vi "DAQmx_Pulse_TrainSlow.vi"(0 "Counter(s)":tag="PXI1Slot3/ctr1", 1 "Start?":bool=TRUE, 3 "FillTime":dbl=20.0 format="%0.2f", 5 "DrainTime":dbl=1.0 min=0.0 format="%0.2f") -> ()   [LabVIEW 2011]
doc: "This VI is set to drive a \"puffer\" valve for pulsed gas releases. It is configured for the stack to be connected to the Normally Open valve port (oddly!)- this is because that port was found to permit higher flow rates. The default logic level has been adjusted accordingly."
uses:
  <vilib>/DAQmx/create/channels.llb/DAQmx Create Channel (CO-Pulse Generation-Time).vi
  <vilib>/DAQmx/configure/timing.llb/DAQmx Timing (Implicit).vi
panel:
  out "error out":errorcluster
  # "For instructions, select Help>>Show Context Help"
  # "Channel Parameters"
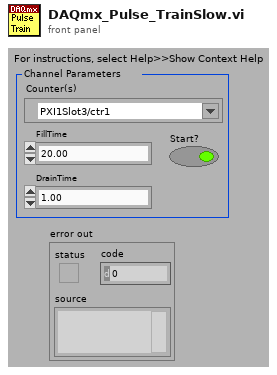
[diagram p1: front panel]
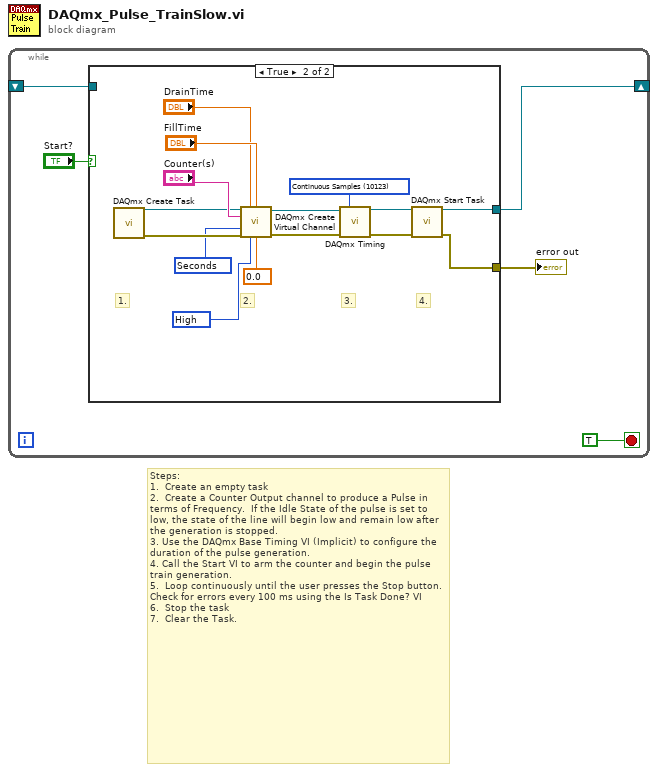
[diagram p0: block diagram]
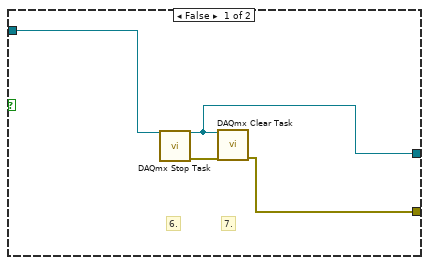
[diagram p2: hidden frame]
diagram:
  # "Steps: \n1.  Create an empty task\n2.  Create a Counter Output channel to produce a Pulse in terms of Frequency.  If the Idle State of the pulse is set to low, the state of the line will begin low and remain low after the generation is stopped.\n3. Use the DAQmx Base Timing VI (Implicit) to configure the duration of the pulse generation.\n4. Call the Start VI to arm the counter and begin the pulse train generation.\n5.  Loop continuously until the user presses the Stop button. Check for errors every 100 ms using the Is Task Done? VI\n6.  Stop the task\n7.  Clear the Task."
  n1 = while {
    shift-right: [w5] -> _
    shift-left: _ -> [w3]
    stop <- TRUE stop-if-true
    n2 = case shown="True" "Start?" {
      tunnel: [w7 w15] -> w5
      tunnel: w3 -> [w8 _]
      tunnel: [w6 w12] -> w1
      frame False {
        # "7."
        # "6."
        n3 = call <vilib>:"DAQmx Stop Task.vi"("task/channels in"=w8) -> ("task out"=w7:refnum<k21>, "error out"=w9:errorcluster)  [unwired: 1 in, 12 out]
        n4 = call <vilib>:"DAQmx Clear Task.vi"("task in"=w7, "error in"=w9) -> ("error out"=w6:errorcluster)  [unwired: 13 out]
      }
      frame True {
        w13 = 10192 items=["High"=10192, "Low"=10214] ("idle state")
        w14 = 10364 items=["Seconds"=10364] ("units")
        w20 = 10123 items=["Finite Samples"=10178, "Continuous Samples"=10123] ("sample mode")
        # "4."
        # "3."
        # "2."
        # "1."
        n5 = call <vilib>:"DAQmx Create Task.vi"() -> ("task out"=w16:refnum<k21>, "error out"=w17:errorcluster)  [unwired: 5 in, 9 out]
        n6 = call-poly <vilib>:"DAQmx Create Virtual Channel.vi"("task in"=w16, "high time"="DrainTime", "low time"="FillTime", "counter"="Counter(s)", "units"=w14, "error in"=w17, "idle state"=w13, "initial delay"=0.0) -> ("task out"=w23:refnum<k21>, "error out"=w24:errorcluster)  [unwired: 1 in, 5 out]
        n7 = call-poly <vilib>:"DAQmx Timing.vi"("task/channels in"=w23, "sample mode"=w20, "error in"=w24) -> ("task out"=w21:refnum<k21>, "error out"=w22:errorcluster)  [unwired: 1 in, 10 out]
        n8 = call <vilib>:"DAQmx Start Task.vi"("task/channels in"=w21, "error in"=w22) -> ("task out"=w15:refnum<k21>, "error out"=w12:errorcluster)  [unwired: 12 out]
      }
    }
    "error out" <- w1
  }
